vi "Switch Shutdown.vi"(8 "error in (no error)":errorcluster, 11 "VISA resource name in":refnum<visa-resource-name>) -> (0 "error out":errorcluster, 3 "VISA resource name out":refnum<visa-resource-name>)   [LabVIEW 2016, in "Hall Effect Library.lvlib"]
uses:
  Hall Effect Library.lvlib
  Global Variables/Instruments.vi
  Switch Shutdown (3706).vi
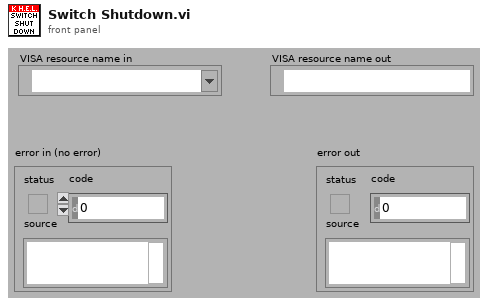
[diagram p1: front panel]
types:
  T1 = typedef "Hall Effect Library.lvlib/Switches.ctl" = enum16{"3706A"}
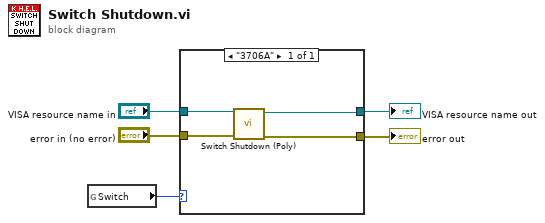
[diagram p0: block diagram]
diagram:
  n1 = global read "Instruments.vi" "Switch"() -> (w5:T1)
  n2 = case shown="\"3706A\"" w5 {
    tunnel: "error in (no error)" -> [w8]
    tunnel: [w6] -> w1
    tunnel: [w7] -> w2
    tunnel: "VISA resource name in" -> [w9]
    frame "3706A" {
      n3 = call-poly "Switch Shutdown (Poly).vi"("error in (no error)"=w8, "VISA resource name in"=w9) -> ("error out"=w6:errorcluster, "VISA resource name out"=w7:refnum<visa-resource-name>)  [unwired: 8 in]
    }
  }
  "error out" <- w1
  "VISA resource name out" <- w2
